vi "Telescope Convert HHMMSS to RA and DEC Angle.vi"(10 "Dec String":string, 11 "RA String":string) -> (1 "RA and DEC":T1, 2 "DEC":dbl, 3 "RA":dbl)   [LabVIEW 2024, in "Telescope.lvclass"]
uses:
  Telescope.lvclass
  typedefs/CC cluster RA and DEC.ctl
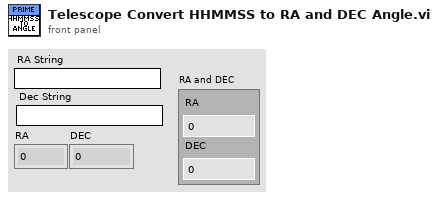
[diagram p1: front panel]
types:
  T1 = typedef "CC cluster RA and DEC.ctl" = cluster{"RA":dbl, "DEC":dbl}
  T2 = typedef "Telescope cluster Dec.ctl" = cluster{"hours":dbl, "Minutes":dbl, "seconds":dbl, "sign":dbl}
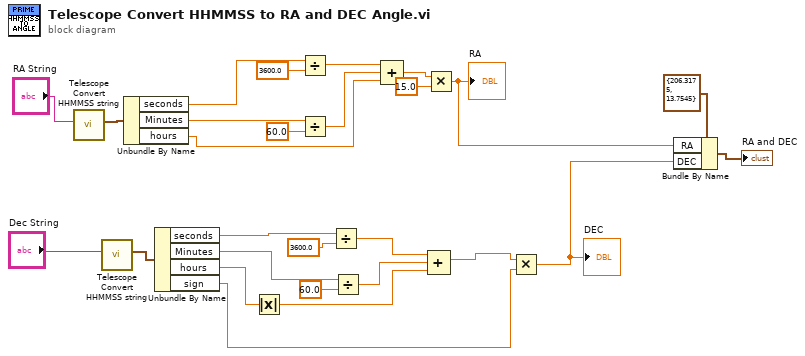
[diagram p0: block diagram]
diagram:
  n1 = call "Telescope Convert HHMMSS string.vi"("RA String"="RA String") -> ("Right Ascension"=w17:T2)  [unwired: 10 in]
  n2 = call "Telescope Convert HHMMSS string.vi"("RA String"="Dec String") -> ("Right Ascension"=w13:T2)  [unwired: 10 in]
  n3 = Unbundle By Name(w17) -> ("seconds"=w16:dbl, "Minutes"=w15:dbl, "hours"=w14:dbl)
  n4 = Unbundle By Name(w13) -> ("seconds"=w12:dbl, "Minutes"=w11:dbl, "hours"=w7:dbl, "sign"=w2:dbl)
  n5 = Absolute Value(x=w7) -> (abs(x)=w8:dbl)
  n6 = Divide(x=w16, y=3600.0) -> (x/y=w25:dbl)
  n7 = Divide(x=w15, y=60.0) -> (x/y=w24:dbl)
  n8 = Divide(x=w12, y=3600.0) -> (x/y=w10:dbl)
  n9 = Divide(x=w11, y=60.0) -> (x/y=w9:dbl)
  n10 = Compound Arithmetic op=ADD(w25, w24, w14) -> (w23:dbl)
  n11 = Multiply(x=w23, y=15.0) -> (x*y=w5:dbl)
  "RA" <- w5
  n12 = Compound Arithmetic op=ADD(w10, w9, w8) -> (w3:dbl)
  n13 = Multiply(x=w3, y=w2) -> (x*y=w1:dbl)
  "DEC" <- w1
  n14 = Bundle By Name(cluster=T1 {"RA"=206.3175, "DEC"=13.7545} ("RA and DEC"), "RA"=w5, "DEC"=w1) -> (→"RA and DEC":T1)
